vi "Save_Table.vi"(8 "Error In":errorcluster, 11 "MAC & Name In":string[][](array[string])) -> (0 "Error Out":errorcluster)   [LabVIEW 2017]
uses:
  <vilib>/Utility/file.llb/Write Delimited Spreadsheet (string).vi
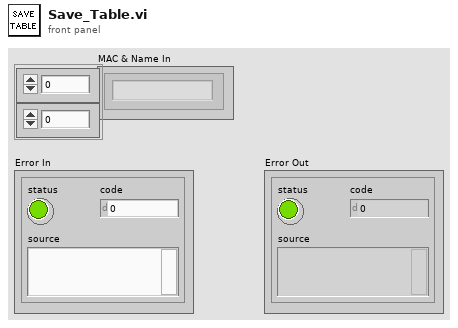
[diagram p1: front panel]
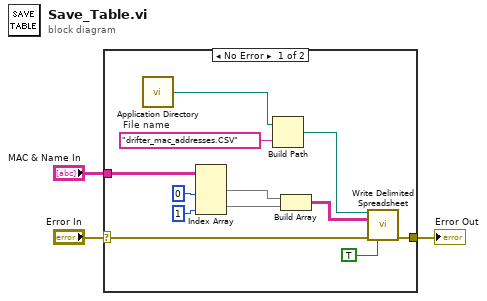
[diagram p0: block diagram]
diagram:
  n1 = case shown="No Error" "Error In" {
    selector: "Error In" -> [w4 w16]
    tunnel: "MAC & Name In" -> [w13 _]
    tunnel: [w5 w16] -> w3
    frame No Error {
      w15 = "drifter_mac_addresses.CSV"  # File name
      n2 = call <vilib>:"Application Directory.vi"() -> ("Application Directory"=w14:path)
      n3 = Index Array(array=w13, index (col) #1=0 ("disabled index (col)"), index (col) #2=1 ("index (col)")) -> (element #1=w12:string[], element #2=w11:string[])  [unwired: 2 in]
      n4 = Build Path(base path=w14, name or relative path=w15) -> (appended path=w8:path)
      n5 = Build Array(w12, w11) -> (w7:string[][])
      n6 = call-poly <vilib>:"Write Delimited Spreadsheet.vi"("file path (dialog if empty)"=w8, "2D data"=w7, "error in (no error)"=w4, "transpose? (no:F)"=TRUE) -> ("error out"=w5:errorcluster)  [unwired: 10 in, 1 out]
    }
    frame Error {
    }
  }
  "Error Out" <- w3
